vi "Write String Data.vi"(10 "String Data":string, 11 "Caller Test Harness in":refnum<class "Caller Test Harness.lvclass">) -> (3 "Caller Test Harness out":refnum<class "Caller Test Harness.lvclass">)   [LabVIEW 2020, in "Caller Test Harness.lvlib" / "Caller Test Harness.lvclass"]
uses:
  Caller Test Harness.lvclass
  <vilib>/ActorFramework/Actor/Actor.lvclass
  <vilib>/ActorFramework/Stop Msg/Stop Msg.lvclass
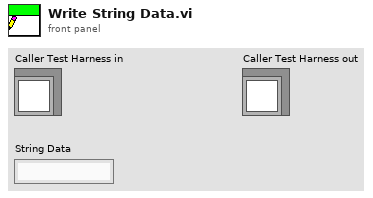
[diagram p1: front panel]
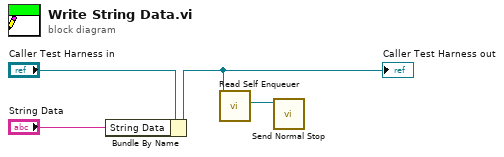
[diagram p0: block diagram]
diagram:
  n1 = Bundle By Name(cluster="Caller Test Harness in", "String Data"="String Data") -> (w2:refnum<class "Caller Test Harness.lvclass">)
  "Caller Test Harness out" <- w2
  n2 = call <vilib>:"Read Self Enqueuer.vi"("Actor"=w2) -> ("Self Enqueuer"=w1:refnum<class "Message Enqueuer.lvclass">)  [unwired: 10 in]
  n3 = call <vilib>:"Send Normal Stop.vi"("Message Enqueuer"=w1) -> ()  [unwired: 10 in, 1 out]
